vi "Measure_dC_dV.vi"(5 "Junction Name":string, 6 "UiDefinition":T1, 7 ".NET Refnum":refnum<k24>, 8 "new file path (Not A Path if cancelled)":path, 10 "appended path":path, 11 ".NET Refnum in":refnum<k24>) -> (0 "error out":errorcluster, 3 "Cluster":cluster{dbl[], dbl[]})   [LabVIEW 2020]
uses:
  UIReferences.ctl
  C:/Users/User/Desktop/Automation/CurrentVersion/LabviewDXFViewer/bin/Release/LabviewDXFViewer.exe
  LabviewDXFViewer/bin/Release/LabviewDXFViewer.exe
  <vilib>/Analysis/6fits.llb/Curve Fitting Criteria.ctl
  <vilib>/Utility/file.llb/Write Delimited Spreadsheet (DBL).vi
  <vilib>/Utility/file.llb/Write Delimited Spreadsheet (string).vi
  <vilib>/Analysis/NI_AALPro.lvlib
panel:
  in  "CurrentPositionIndex":i32
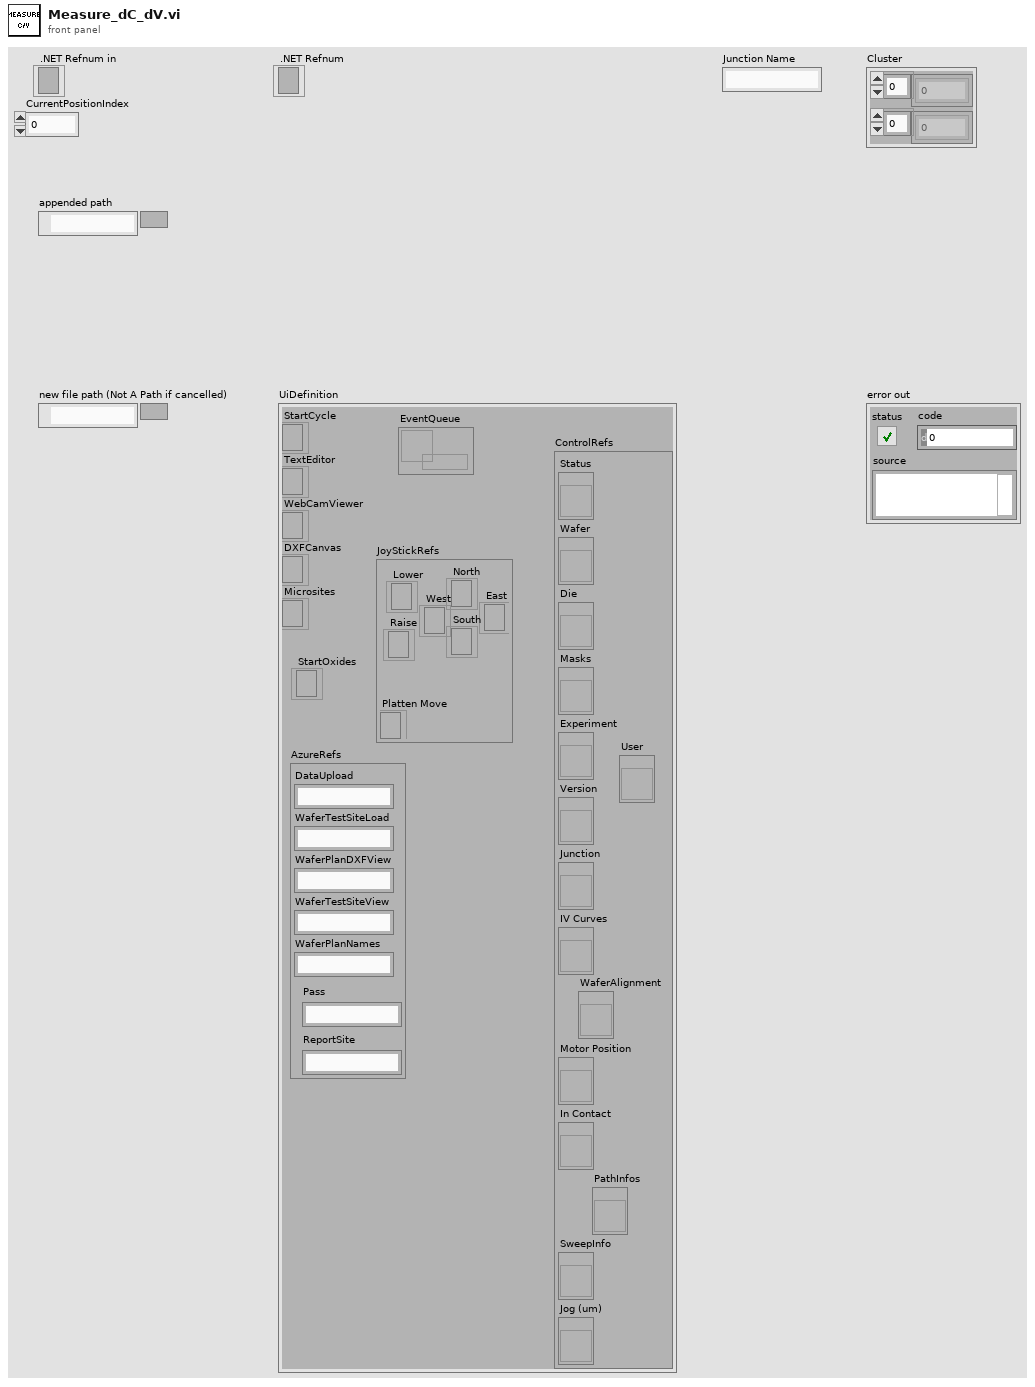
[diagram p1: front panel]
types:
  T1 = typedef "UIReferences.ctl" = cluster{"StartCycle":refnum<k24>, "TextEditor":refnum<k24>, "WebCamViewer":refnum<k24>, "DXFCanvas":refnum<k24>, "Microsites":refnum<k24>, "JoyStickRefs":cluster{"North":refnum<k24>, "Lower":refnum<k24>, "Raise":refnum<k24>, "Platten Move":refnum<k24>, "West":refnum<k24>, "East":refnum<k24>, "South":refnum<k24>}, "AzureRefs":cluster{"DataUpload":string, "WaferTestSiteLoad":string, "WaferPlanDXFView":string, "WaferTestSiteView":string, "WaferPlanNames":string, "Pass":string, "ReportSite":string}, "ControlRefs":cluster{"Status":refnum<vi>, "Wafer":refnum<vi>, "Die":refnum<vi>, "Masks":refnum<vi>, "Experiment":refnum<vi>, "Version":refnum<vi>, "Junction":refnum<vi>, "IV Curves":refnum<vi>, "Motor Position":refnum<vi>, "In Contact":refnum<vi>, "SweepInfo":refnum<vi>, "Jog (um)":refnum<vi>, "PathInfos":refnum<vi>, "User":refnum<vi>, "WaferAlignment":refnum<vi>}, "EventQueue":refnum<queue>, "StartOxides":refnum<k24>}
  T2 = typedef "NI_AALPro.lvlib/Curve Fitting Criteria.ctl" = u16
  T3 = typedef "CapacitanceInfos.ctl" = cluster{"Conductance":dbl, "CapacitanceIV":dbl, "Intercept":dbl, "CapacitanceSW":dbl, "Sum":dbl, "CapacitanceInfos":T4[], "CapacitancePhase":dbl, "dC/dV":dbl, "Function":string, "OtherInfo":dbl[][]}
  T4 = typedef "CapacitanceRecord.ctl" = cluster{"Freq":dbl, "Vpp":dbl, "PhaseS":dbl, "Irms":dbl, "PhaseC":dbl, "Theta":dbl, "VDrive":dbl, "Capacitance":dbl, "Other":dbl}
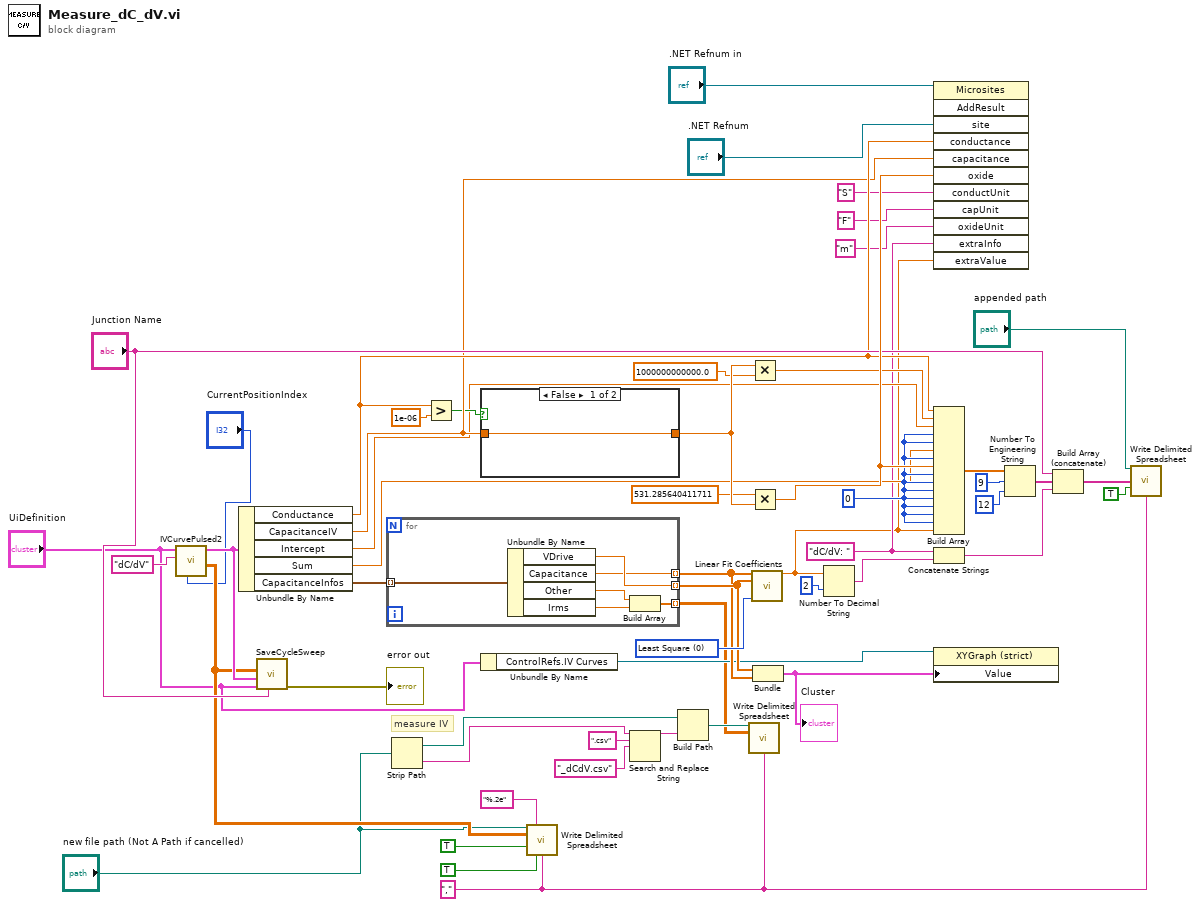
[diagram p0: block diagram]
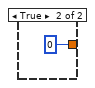
[diagram p2: hidden frame]
diagram:
  w3 = "dC/dV: "
  w8 = "," ("delimiter (\\t)")
  w51 = T2 0 items=["Least Square", "Least Absolute Residual", "Bisquare"] ("method")
  w48 = 0
  # "measure IV"
  n1 = call "IVCurvePulsed2.vi"("CurrentPositionIndex"="CurrentPositionIndex", "Program"="dC/dV", "UiDefinition"="UiDefinition") -> ("appended array"=w27:dbl[][], "InfoCluster"=w40:T3)  [unwired: 7 in]
  n2 = Unbundle By Name(w40) -> ("Conductance"=w42:dbl, "CapacitanceIV"=w41:dbl, "Intercept"=w30:dbl, "Sum"=w31:dbl, "CapacitanceInfos"=w43:T4[])
  n3 = call "SaveCycleSweep.vi"("JunctionName"="Junction Name", "UiDefinition 2"="UiDefinition", "InfoCluster"=w40, "appended array"=w27) -> ("error out"=→"error out":errorcluster)  [unwired: 7 in]
  n4 = for {
    tunnel: w43 -> [w60] mode=indexing
    tunnel: [w59] -> w50 mode=indexing
    tunnel: [w58] -> w49 mode=indexing
    tunnel: [w57] -> w7 mode=indexing
    n5 = Unbundle By Name(w60) -> ("VDrive"=w59:dbl, "Capacitance"=w58:dbl, "Other"=w56:dbl, "Irms"=w55:dbl)
    n6 = Build Array(w56, w55) -> (w57:dbl[])
  }
  n7 = Strip Path(path="new file path (Not A Path if cancelled)") -> (stripped path=w14:path, name=w18:string)
  n8 = Greater?(x=w42, y=1e-06) -> (0:w34:bool)
  n9 = case shown="False" w34 {
    tunnel: [w61 0] -> w53
    tunnel: w41 -> [w61 _]
    frame False {
    }
    frame True {
    }
  }
  n10 = Unbundle By Name("UiDefinition") -> ("ControlRefs.IV Curves"=w13:refnum<vi>)
  n11 = call-poly <vilib>:"Write Delimited Spreadsheet.vi"("file path (dialog if empty)"="new file path (Not A Path if cancelled)", "format (%.3f)"="%.2e", "2D data"=w27, "append to file? (new file:F)"=TRUE, "transpose? (no:F)"=TRUE, "delimiter (\\t)"=w8) -> ()  [unwired: 8 in, 2 out]
  n12 = Search and Replace String(input string=w18, search string=".csv", replace string="_dCdV.csv" ("replace string (\"\")")) -> (result string=w15:string)  [unwired: 5 in, 3 out]
  n13 = Build Path(base path=w14, name or relative path=w15) -> (appended path=w9:path)
  n14 = call-poly <vilib>:"Write Delimited Spreadsheet.vi"("file path (dialog if empty)"=w9, "2D data"=w7, "delimiter (\\t)"=w8) -> ()  [unwired: 11 in, 2 out]
  n15 = Multiply(x=w53, y=1000000000000.0) -> (x*y=w32:dbl)
  n16 = Multiply(x=531.285640411711, y=w53) -> (x*y=w54:dbl)
  n17 = call <vilib>:"Linear Fit Coefficients.vi"("Y"=w49, "X"=w50, "method"=w51) -> ("slope"=w2:dbl)  [unwired: 10 in, 2 out]
  n18 = Bundle(w50, w49) -> (w11:cluster{dbl[], dbl[]})  [unwired: 1 in]
  "Cluster" <- w11
  n19 = Number To Decimal String(number=w2, width (-)=i16 2) -> (decimal integer string=w6:string)
  n20 = invoke class="Microsites" method="AddResult"(reference=".NET Refnum in", "site"=".NET Refnum", "conductance"=w42, "capacitance"=w41, "oxide"=w54, "conductUnit"="S", "capUnit"="F", "oxideUnit"="m" ("interceptUnit"), "extraInfo"=w3, "extraValue"=w2) -> ()  [unwired: 2 in, 12 out]
  n21 = Build Array(w42, w32, w30, w48, w48, w31, w48, w54, w48, w48, w48, w48, w48, w48, w48, w2) -> (w29:dbl[])
  n22 = Concatenate Strings(w3, w6) -> (w4:string)
  n23 = property class="XYGraph (strict)"(reference=w13, "Value"=w11) -> ()  [unwired: 1 in, 2 out]
  n24 = Number To Engineering String(2:i16 12 ("precision (6)"), 3:i16 9 ("width (-)"), 4:w29) -> (0:w21:string[])  [unwired: 1 in]
  n25 = Build Array (concatenate)("Junction Name", w21, w4) -> (w23:string[])
  n26 = call-poly <vilib>:"Write Delimited Spreadsheet.vi"("file path (dialog if empty)"="appended path", "1D data"=w23, "append to file? (new file:F)"=TRUE, "delimiter (\\t)"=w8) -> ()  [unwired: 10 in, 2 out]
